vi "Procedura abilitazione potenza.vi"(9 "All Data":T3 {"MISURE ALL"."Cluster READ NI"."AI (4-20mA)"."AI 15" format="%#_6f"; "MISURE ALL"."Cluster READ NI"."AI (4-20mA)"."AI 14" format="%#_6f"; "MISURE ALL"."Cluster READ NI"."AI (4-20mA)"."AI 13" format="%#_6f"; "MISURE ALL"."Cluster READ NI"."AI (4-20mA)"."AI 11" format="%#_6f"; "MISURE ALL"."Cluster READ NI"."AI (4-20mA)"."AI 10" format="%#_6f"; "MISURE ALL"."Cluster READ NI"."AI (4-20mA)"."AI 9" format="%#_6f"; "MISURE ALL"."Cluster READ NI"."AI (4-20mA)"."AI 4" format="%#_6f"; "MISURE ALL"."Cluster READ NI"."AI (4-20mA)"."AI 12" format="%#_6f"; "MISURE ALL"."Cluster READ NI"."AI (4-20mA)"."AI 0" format="%#_6f"; "MISURE ALL"."Cluster READ NI"."AI (4-20mA)"."AI 1" format="%#_6f"; "MISURE ALL"."Cluster READ NI"."AI (4-20mA)"."AI 2" format="%#_6f"; "MISURE ALL"."Cluster READ NI"."AI (4-20mA)"."AI 3" format="%#_6f"; "MISURE ALL"."Cluster READ NI"."AI (4-20mA)"."AI 5" format="%#_6f"; "MISURE ALL"."Cluster READ NI"."AI (4-20mA)"."AI 6" format="%#_6f"; "MISURE ALL"."Cluster READ NI"."AI (4-20mA)"."AI 7" format="%#_6f"; "MISURE ALL"."Cluster READ NI"."AI (4-20mA)"."AI 8" format="%#_6f"; "MISURE ALL"."Cluster READ NI"."AI (0-10V)"."AI 31" format="%#_6f"; "MISURE ALL"."Cluster READ NI"."AI (0-10V)"."AI 30" format="%#_6f"; "MISURE ALL"."Cluster READ NI"."AI (0-10V)"."AI 29" format="%#_6f"; "MISURE ALL"."Cluster READ NI"."AI (0-10V)"."AI 28" format="%#_6f"; "MISURE ALL"."Cluster READ NI"."AI (0-10V)"."AI 27" format="%#_6f"; "MISURE ALL"."Cluster READ NI"."AI (0-10V)"."AI 26" format="%#_6f"; "MISURE ALL"."Cluster READ NI"."AI (0-10V)"."AI 25" format="%#_6f"; "MISURE ALL"."Cluster READ NI"."AI (0-10V)"."AI 24" format="%#_6f"; "MISURE ALL"."Cluster READ NI"."AI (0-10V)"."AI 23" format="%#_6f"; "MISURE ALL"."Cluster READ NI"."AI (0-10V)"."AI 22" format="%#_6f"; "MISURE ALL"."Cluster READ NI"."AI (0-10V)"."AI 21" format="%#_6f"; "MISURE ALL"."Cluster READ NI"."AI (0-10V)"."AI 20" format="%#_6f"; "MISURE ALL"."Cluster READ NI"."AI (0-10V)"."AI 19" format="%#_6f"; "MISURE ALL"."Cluster READ NI"."AI (0-10V)"."AI 18" format="%#_6f"; "MISURE ALL"."Cluster READ NI"."AI (0-10V)"."AI 17" format="%#_6f"; "MISURE ALL"."Cluster READ NI"."AI (0-10V)"."AI 16" format="%#_6f"; "MISURE ALL"."Cluster READ NI"."AI (0-10V)"."AI 15" format="%#_6f"; "MISURE ALL"."Cluster READ NI"."AI (0-10V)"."AI 14" format="%#_6f"; "MISURE ALL"."Cluster READ NI"."AI (0-10V)"."AI 13" format="%#_6f"; "MISURE ALL"."Cluster READ NI"."AI (0-10V)"."AI 11" format="%#_6f"; "MISURE ALL"."Cluster READ NI"."AI (0-10V)"."AI 10" format="%#_6f"; "MISURE ALL"."Cluster READ NI"."AI (0-10V)"."AI 9" format="%#_6f"; "MISURE ALL"."Cluster READ NI"."AI (0-10V)"."AI 4" format="%#_6f"; "MISURE ALL"."Cluster READ NI"."AI (0-10V)"."AI 12" format="%#_6f"; "MISURE ALL"."Cluster READ NI"."AI (0-10V)"."AI 0" format="%#_6f"; "MISURE ALL"."Cluster READ NI"."AI (0-10V)"."AI 1" format="%#_6f"; "MISURE ALL"."Cluster READ NI"."AI (0-10V)"."AI 2" format="%#_6f"; "MISURE ALL"."Cluster READ NI"."AI (0-10V)"."AI 3" format="%#_6f"; "MISURE ALL"."Cluster READ NI"."AI (0-10V)"."AI 5" format="%#_6f"; "MISURE ALL"."Cluster READ NI"."AI (0-10V)"."AI 6" format="%#_6f"; "MISURE ALL"."Cluster READ NI"."AI (0-10V)"."AI 7" format="%#_6f"; "MISURE ALL"."Cluster READ NI"."AI (0-10V)"."AI 8" format="%#_6f"}, 10 "Impostazioni elettriche in":T1, 11 "Stato":string) -> (0 "This VI":refnum<vi>, 2 "Fine step":bool, 3 "stato out":string)   [LabVIEW 2019]
uses:
  TypeDef/Cluster MISURE.ctl
  TypeDef/MISURE NM.ctl
  TypeDef/Cluster misure ALL.ctl
  TypeDef/Cluster NI.ctl
  cDAQ_PLC Folder/controls/StatoAO_cdaq.ctl
  cDAQ_PLC Folder/controls/statoDO_Cdaq.ctl
  TypeDef/MISURE WT.ctl
  TypeDef/ClusterRes.ctl
  TypeDef/INTERFACCIA.ctl
  TypeDef/Lista AO sistema.ctl
  TypeDef/DOinterfaccia.ctl
  cDAQ_PLC Folder/ST1200_LIST_IO/STATO PLC 1.ctl
  cDAQ_PLC Folder/ST1200_LIST_IO/Uscite PLC 1.ctl
  cDAQ_PLC Folder/controls/statoAO_plc_1.ctl
  cDAQ_PLC Folder/ST1200_LIST_IO/StatoDO_PLC_1.ctl
  SINUS PENTA SANTERNO/controls/Parametri inverter letti.ctl
  cDAQ_PLC Folder/ST1200_LIST_IO/STATO PLC 2.ctl
  cDAQ_PLC Folder/ST1200_LIST_IO/Uscite PLC 2.ctl
  cDAQ_PLC Folder/controls/statoAO_plc_2.ctl
  cDAQ_PLC Folder/ST1200_LIST_IO/StatoDO_PLC_2.ctl
  cDAQ_PLC Folder/ST1200_LIST_IO/STATO PLC 3.ctl
  cDAQ_PLC Folder/ST1200_LIST_IO/Uscite PLC 3.ctl
  cDAQ_PLC Folder/controls/statoAO_plc_3.ctl
  cDAQ_PLC Folder/ST1200_LIST_IO/StatoDO_PLC_3.ctl
  DCREG/Parametri DCREG letti.ctl
  TypeDef/Impostazioni elettriche.ctl
  TypeDef/Collegamenti_elettrici.ctl
  cDAQ_PLC Folder/cDAQ/SET ARRAY DO.ctl
  cDAQ_PLC Folder/cDAQ/SET SINGLE DO.ctl
  cDAQ_PLC Folder/cDAQ/DO List.ctl
  Stato alimentatore 1.vi
  Stato comandi freno.vi
  Global allarmi procedure.vi
panel:
  out "Stato 2":string
  out "Abilita freno":bool caption="ABILITA BANCO FRENO \\ ALIMENTATORE"
  in  "OK Button":bool
  out "String":string
  out "RESET CENTRALINA":bool caption="RESET CENTRALINA PROTEZIONI"
  out "Chiusura teleruttore":bool caption="CHIUSURA TELERUTTORE DI POTENZA"
  out "abilitazione elettroserrature":bool caption="ABILITAZIONE ELETTROSERRATURE"
  out "Verifica protezioni chiuse":bool caption="VERIFICA PROTEZIONI CHIUSE"
  # "ABILITAZIONE TELERUTTORE DI POTENZA IN CORSO. \n                               >>ATTENDI<<"
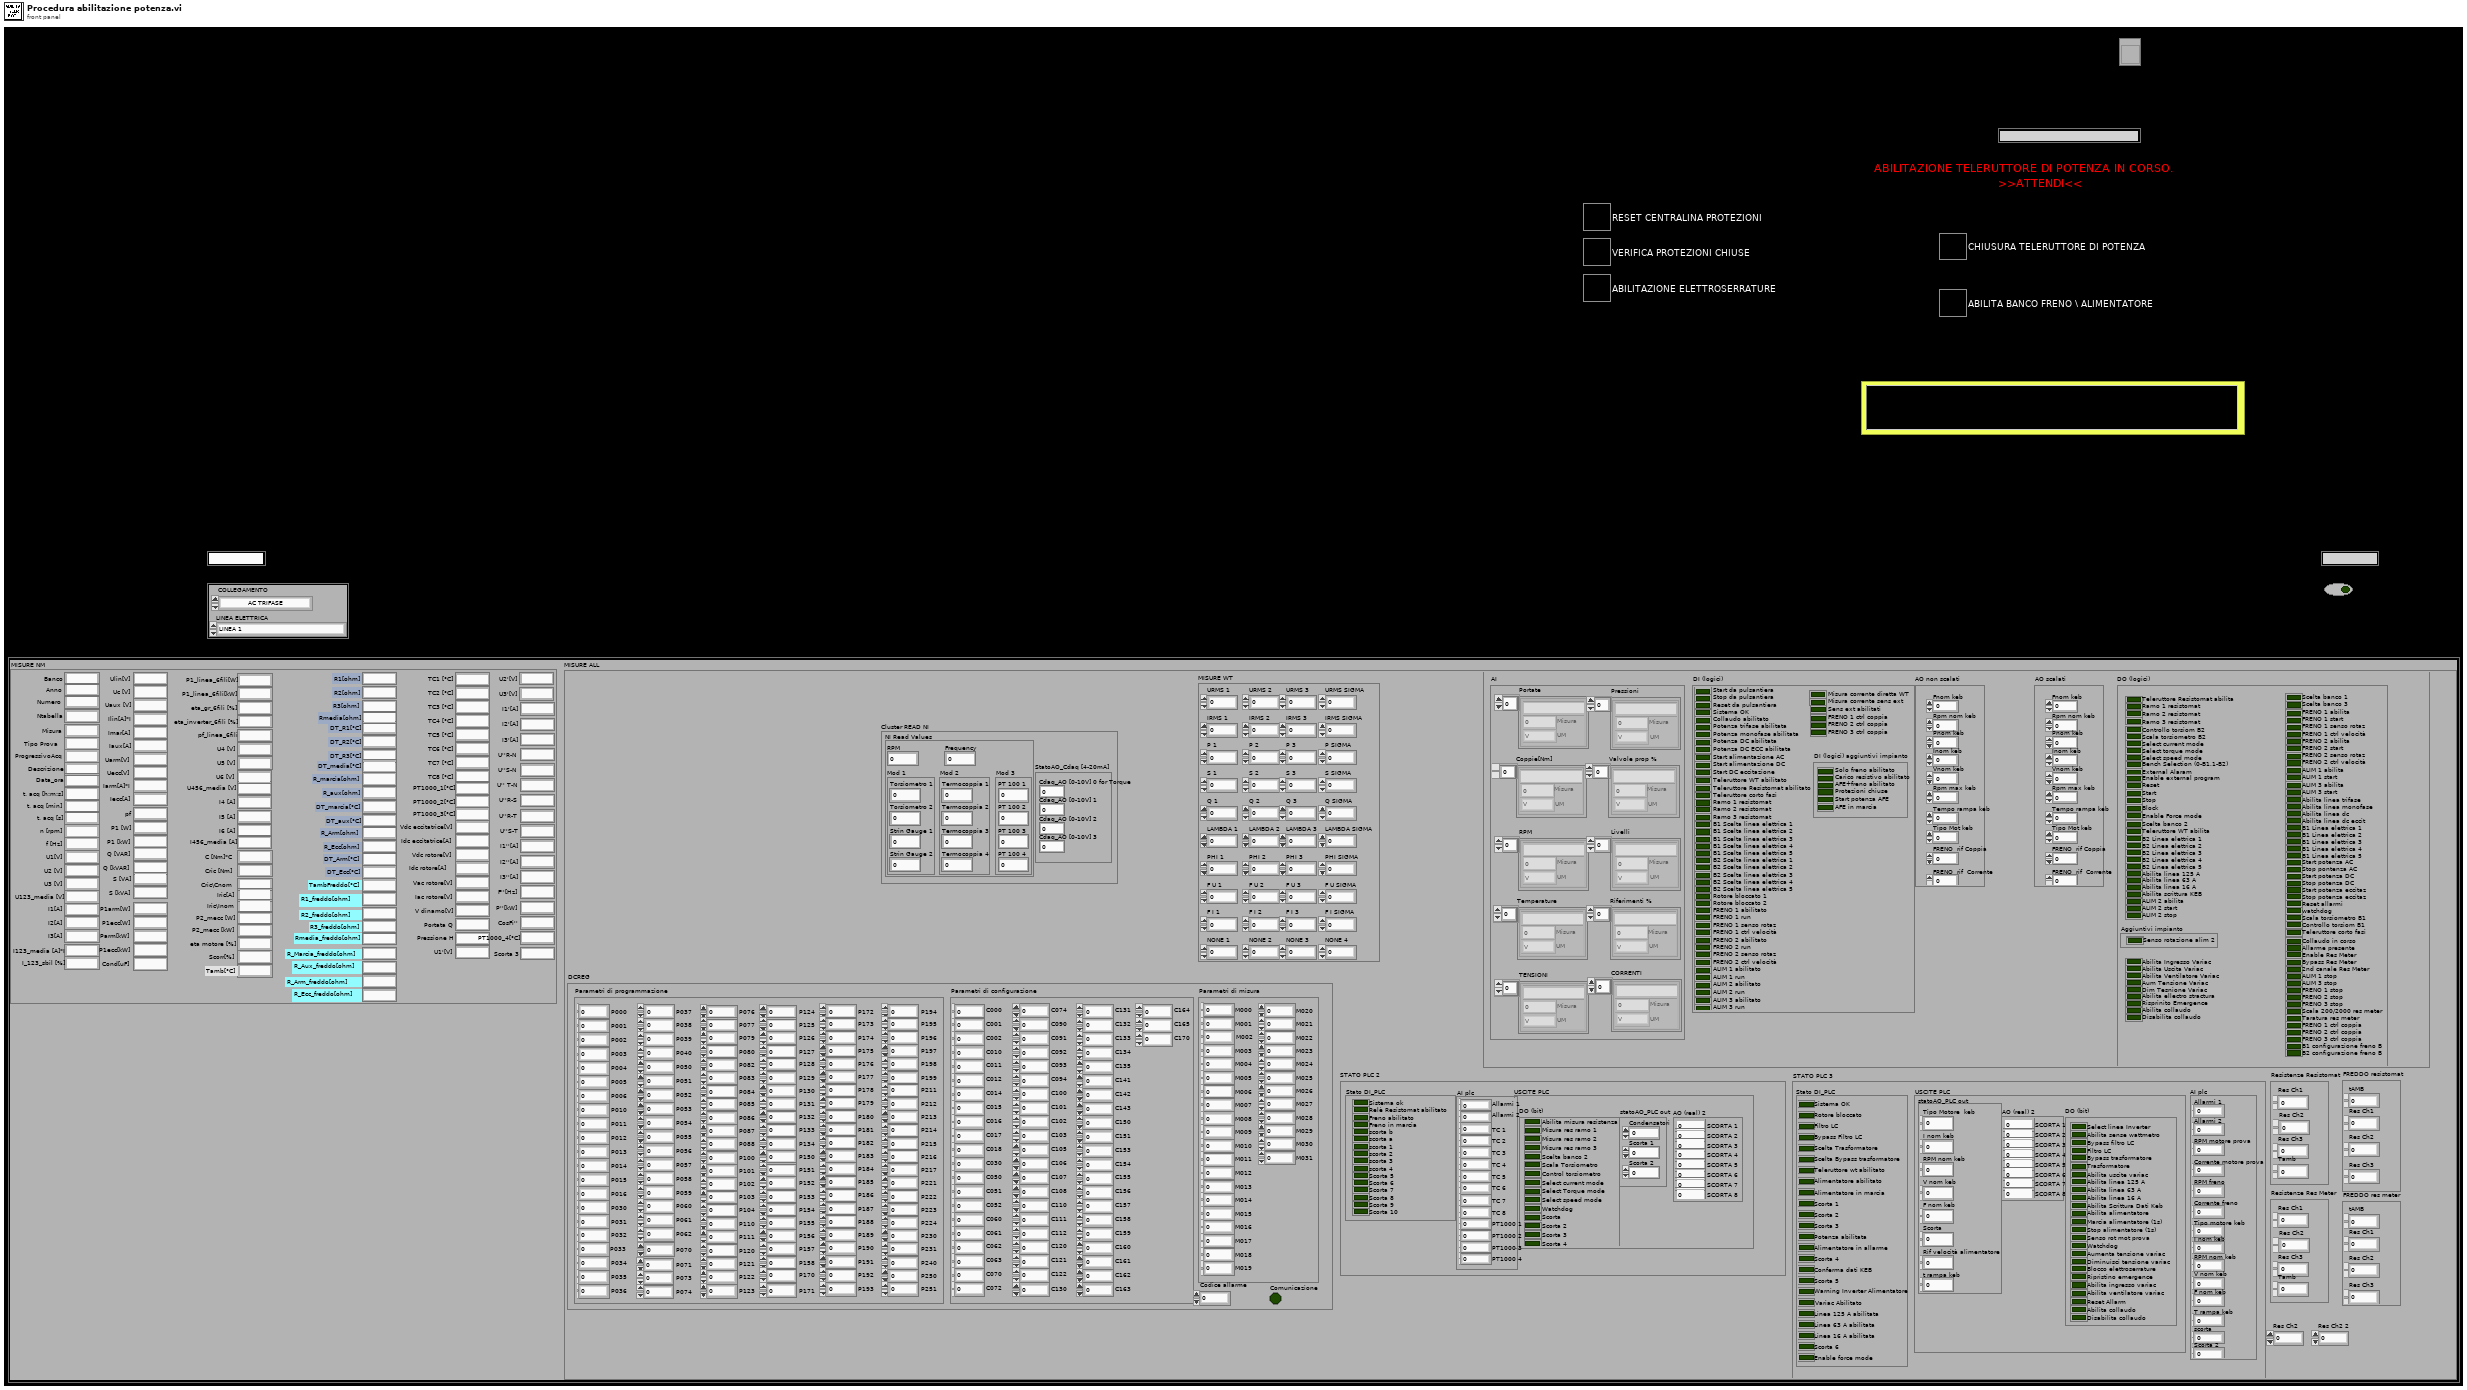
[diagram p1: front panel]
types:
  T1 = typedef "Impostazioni elettriche.ctl" = cluster{"COLLEGAMENTO":T2, "LINEA ELETTRICA":enum16{"LINEA 1", "LINEA 2", "LINEA 3", "LINEA 4", "LINEA 5"}}
  T2 = typedef "Collegamenti_elettrici.ctl" = enum16{"AC TRIFASE", "AC TRIFASE + FRENO", "AC MONOFASE", "DC CON ECCITAZIONE", "DC CON ECCITAZIONE + FRENO", "DC NO ECCITAZIONE", "DC NO ECCITAZIONE + FRENO", "FRENO TRASC + AFE", "SOLO FRENO", "CARICO RESISTIVO", "GENERICO", "SOLO ACQUISITORE", "SCORTA 4", "SCORTA 5", "SCORTA 6"}
  T3 = typedef "Cluster MISURE.ctl" = cluster{"MISURE NM":T4, "MISURE ALL":T5}
  T4 = typedef "MISURE NM.ctl" = cluster{"Banco":string, "Anno":string, "Numero":string, "Ntabella":string, "Misura":string, "Tipo Prova":string, "ProgressivoAcq":string, "Descrizione":string, "Data_ora":string, "t. acq [h:m:s]":string, "t. acq [min]":string, "t. acq [s]":string, "n [rpm]":string, "f [Hz]":string, "U1[V]":string, "U2 [V]":string, "U3 [V]":string, "U123_media [V]":string, "I1[A]":string, "I2[A]":string, "I3[A]":string, "I123_media [A]*I":string, "I_123_sbil [%]":string, "Ulin[V]":string, "Uc [V]":string, "Uaux [V]":string, "Ilin[A]*I":string, "Imar[A]":string, "Iaux[A]":string, "Uarm[V]":string, "Uecc[V]":string, "Iarm[A]*I":string, "Iecc[A]":string, "pf":string, "P1 [W]":string, "P1 [kW]":string, "Q [VAR]":string, "Q [kVAR]":string, "S [VA]":string, "S [kVA]":string, "P1arm[W]":string, "P1ecc[W]":string, "Parm[kW]":string, "P1ecc[kW]":string, "Cond[uF]":string, "P1_linea_6fili[W]":string, "P1_linea_6fili[kW]":string, "eta_gr_6fili [%]":string, "eta_inverter_6fili [%]":string, "pf_linea_6fili":string, "U4 [V]":string, "U5 [V]":string, "U6 [V]":string, "U456_media [V]":string, "I4 [A]":string, "I5 [A]":string, "I6 [A]":string, "I456_media [A]":string, "C [Nm]*C":string, "Cric [Nm]":string, "Cric\\Cnom":string, "Iric[A]":string, "Iric\\Inom":string, "P2_mecc [W]":string, "P2_mecc [kW]":string, "eta motore [%]":string, "Scorr[%]":string, "Tamb[°C]":string, "R1[ohm]":string, "R2[ohm]":string, "R3[ohm]":string, "Rmedia[ohm]":string, "DT_R1[°C]":string, "DT_R2[°C]":string, "DT_R3[°C]":string, "DT_media[°C]":string, "R_marcia[ohm]":string, "R_aux[ohm]":string, "DT_marcia[°C]":string, "DT_aux[°C]":string, "R_Arm[ohm]":string, "R_Ecc[ohm]":string, "DT_Arm[°C]":string, "DT_Ecc[°C]":string, "TambFreddo[°C]":string, "R1_freddo[ohm]":string, "R2_freddo[ohm]":string, "R3_freddo[ohm]":string, "Rmedia_freddo[ohm]":string, "R_Marcia_freddo[ohm]":string, "R_Aux_freddo[ohm]":string, "R_Arm_freddo[ohm]":string, "R_Ecc_freddo[ohm]":string, "TC1 [°C]":string, "TC2 [°C]":string, "TC3 [°C]":string, "TC4 [°C]":string, "TC5 [°C]":string, "TC6 [°C]":string, "TC7 [°C]":string, "TC8 [°C]":string, "PT1000_1[°C]":string, "PT1000_2[°C]":string, "PT1000_3[°C]":string, "Vdc eccitatrice[V]":string, "Idc eccitatrice[A]":string, "Vdc rotore[V]":string, "Idc rotore[A]":string, "Vac rotore[V]":string, "Iac rotore[V]":string, "V dinamo[V]":string, "Portata Q":string, "Pressione H":string, "U1'[V]":string, "U2'[V]":string, "U3'[V]":string, "I1'[A]":string, "I2'[A]":string, "I3'[A]":string, "U''R-N":string, "U''S-N":string, "U'' T-N":string, "U''R-S":string, "U''R-T":string, "U''S-T":string, "I1''[A]":string, "I2''[A]":string, "I3''[A]":string, "F''[Hz]":string, "P''[kW]":string, "CosFi''":string, "PT1000_4[°C]":string, "Scorta 3":string}
  T5 = typedef "Cluster misure ALL.ctl" = cluster{"Cluster READ NI":T6, "MISURE WT":T9, "Resistenze Resistomat":T10, "INTERFACCIA":T11, "FREDDO resistomat":cluster{"Res Ch1":dbl, "Res Ch2":dbl, "tAMB":dbl, "Res Ch3":dbl}, "STATO PLC 1":T16, "Res Ch2":dbl, "Res Ch2 2":dbl, "FREDDO res meter":cluster{"Res Ch1":dbl, "Res Ch2":dbl, "tAMB":dbl, "Res Ch3":dbl}, "Resistenze Res Meter":T10, "READ SINUS PENTA":T20, "STATO PLC 2":T21, "STATO PLC 3":T25, "DCREG":T29}
  T6 = typedef "Cluster NI.ctl" = cluster{"AI (0-10V)":cluster{"AI 0":dbl, "AI 1":dbl, "AI 2":dbl, "AI 3":dbl, "AI 4":dbl, "AI 5":dbl, "AI 6":dbl, "AI 7":dbl, "AI 8":dbl, "AI 9":dbl, "AI 10":dbl, "AI 11":dbl, "AI 12":dbl, "AI 13":dbl, "AI 14":dbl, "AI 15":dbl, "AI 16":dbl, "AI 17":dbl, "AI 18":dbl, "AI 19":dbl, "AI 20":dbl, "AI 21":dbl, "AI 22":dbl, "AI 23":dbl, "AI 24":dbl, "AI 25":dbl, "AI 26":dbl, "AI 27":dbl, "AI 28":dbl, "AI 29":dbl, "AI 30":dbl, "AI 31":dbl}, "StatoAO_Cdaq[0-10V]":cluster{"AO 1":dbl, "AO 2":dbl, "AO 3":dbl, "AO 4":dbl}, "Contatori [rpm]":cluster{"RPM 1":dbl, "RPM 2":dbl}, "StatoAO_Cdaq [4-20mA]":T7, "StatoDO_Cdaq":T8, "DI":cluster{"Scorta 0":bool, "Scorta 1":bool, "Scorta 2":bool, "Scorta 3":bool, "Scorta 4":bool, "Scorta 5":bool, "Scorta 6":bool, "Scorta 7":bool, "Scorta 8":bool, "Scorta 9":bool, "Scorta 10":bool, "Scorta 11":bool, "Scorta 12":bool, "Scorta 13":bool, "Scorta 14":bool, "Scorta 15":bool, "Scorta 16":bool, "Scorta 17":bool, "Scorta 18":bool, "Scorta 19":bool, "Scorta 20":bool, "Scorta 21":bool, "Scorta 22":bool, "Scorta 23":bool, "Scorta 24":bool, "Scorta 25":bool, "Scorta 26":bool, "Scorta 27":bool, "Scorta 28":bool, "Scorta 29":bool, "Scorta 30":bool, "Scorta 31":bool}, "AI (4-20mA)":cluster{"AI 0":dbl, "AI 1":dbl, "AI 2":dbl, "AI 3":dbl, "AI 4":dbl, "AI 5":dbl, "AI 6":dbl, "AI 7":dbl, "AI 8":dbl, "AI 9":dbl, "AI 10":dbl, "AI 11":dbl, "AI 12":dbl, "AI 13":dbl, "AI 14":dbl, "AI 15":dbl}, "TC [°C]":cluster{"tc 1":dbl, "tc 2":dbl, "tc 3":dbl, "tc 4":dbl}, "NI Read Values":cluster{"RPM":dbl, "Frequency":dbl, "Mod 1":cluster{"Torsiometro 1":dbl, "Torsiometro 2":dbl, "Strin Gauge 1":dbl, "Strin Gauge 2":dbl}, "Mod 2":cluster{"Termocoppia 1":dbl, "Termocoppia 2":dbl, "Termocoppia 3":dbl, "Termocoppia 4":dbl}, "Mod 3":cluster{"PT 100 1":dbl, "PT 100 2":dbl, "PT 100 3":dbl, "PT 100 4":dbl}}}
  T7 = typedef "StatoAO_cdaq.ctl" = cluster{"Cdaq_AO [0-10V] 0 for Torque":dbl, "Cdaq_AO [0-10V] 1":dbl, "Cdaq_AO [0-10V] 2":dbl, "Cdaq_AO [0-10V] 3":dbl}
  T8 = typedef "statoDO_Cdaq.ctl" = cluster{"Scorta 0":bool, "Scorta 1":bool, "Scorta 2":bool, "Scorta 3":bool, "Scorta 4":bool, "Scorta 5":bool, "Scorta 6":bool, "Scorta 7":bool, "Scorta 8":bool, "Scorta 9":bool, "Scorta 10":bool, "Scorta 11":bool, "Scorta 12":bool, "Scorta 13":bool, "Scorta 14":bool, "Scorta 15":bool, "Scorta 16":bool, "Scorta 17":bool, "Scorta 18":bool, "Scorta 19":bool, "Scorta 20":bool, "Scorta 21":bool, "Scorta 22":bool, "Scorta 23":bool, "Scorta 24":bool, "Scorta 25":bool, "Scorta 26":bool, "Scorta 27":bool, "Scorta 28":bool, "Scorta 29":bool, "Scorta 30":bool, "Scorta 31":bool}
  T9 = typedef "MISURE WT.ctl" = cluster{"URMS 1":dbl, "IRMS 1":dbl, "P 1":dbl, "S 1":dbl, "Q 1":dbl, "LAMBDA 1":dbl, "PHI 1":dbl, "F U 1":dbl, "F I 1":dbl, "NONE 1":dbl, "URMS 2":dbl, "IRMS 2":dbl, "P 2":dbl, "S 2":dbl, "Q 2":dbl, "LAMBDA 2":dbl, "PHI 2":dbl, "F U 2":dbl, "F I 2":dbl, "NONE 2":dbl, "URMS 3":dbl, "IRMS 3":dbl, "P 3":dbl, "S 3":dbl, "Q 3":dbl, "LAMBDA 3":dbl, "PHI 3":dbl, "F U 3":dbl, "F I 3":dbl, "NONE 3":dbl, "URMS SIGMA":dbl, "IRMS SIGMA":dbl, "P SIGMA":dbl, "S SIGMA":dbl, "Q SIGMA":dbl, "LAMBDA SIGMA":dbl, "PHI SIGMA":dbl, "F U SIGMA":dbl, "F I SIGMA":dbl, "NONE 4":dbl}
  T10 = typedef "ClusterRes.ctl" = cluster{"Res Ch1":dbl, "Res Ch2":dbl, "Res Ch3":dbl, "Tamb":dbl}
  T11 = typedef "INTERFACCIA.ctl" = cluster{"AI":cluster{"Portate":T12[], "Pressioni":T12[], "Coppie[Nm]":T12[], "Valvole prop %":T12[], "RPM":T12[], "Livelli":T12[], "Temperature":T12[], "Riferimenti %":T12[], "TENSIONI":T12[], "CORRENTI":T12[]}, "DI (logici)":cluster{"Start da pulsantiera":bool, "Stop da pulsantiera":bool, "Reset da pulsantiera":bool, "Sistema OK":bool, "Collaudo abilitato":bool, "Potenza trifase abilitata":bool, "Potenza monofase abilitata":bool, "Potenza DC abilitata":bool, "Potenza DC ECC abilitata":bool, "Start alimentazione AC":bool, "Start alimentazione DC":bool, "Start DC eccitazione":bool, "Teleruttore WT abilitato":bool, "Teleruttore Resistomat abilitato":bool, "Teleruttore corto fasi":bool, "Ramo 1 resistomat":bool, "Ramo 2 resistomat":bool, "Ramo 3 resistomat":bool, "B1 Scelta linea elettrica 1":bool, "B1 Scelta linea elettrica 2":bool, "B1 Scelta linea elettrica 3":bool, "B1 Scelta linea elettrica 4":bool, "B1 Scelta linea elettrica 5":bool, "B2 Scelta linea elettrica 1":bool, "B2 Scelta linea elettrica 2":bool, "B2 Scelta linea elettrica 3":bool, "B2 Scelta linea elettrica 4":bool, "B2 Scelta linea elettrica 5":bool, "Rotore bloccato 1":bool, "Rotore bloccato 2":bool, "FRENO 1 abilitato":bool, "FRENO 1 run":bool, "FRENO 1 senso rotaz":bool, "FRENO 1 ctrl velocità":bool, "FRENO 2 abilitato":bool, "FRENO 2 run":bool, "FRENO 2 senso rotaz":bool, "FRENO 2 ctrl velocità":bool, "ALIM 1 abilitato":bool, "ALIM 1 run":bool, "ALIM 2 abilitato":bool, "ALIM 2 run":bool, "ALIM 3 abilitato":bool, "ALIM 3 run":bool, "FRENO 1 ctrl coppia":bool, "FRENO 2 ctrl coppia":bool, "FRENO 3 ctrl coppia":bool, "DI (logici) aggiuntivi impianto":cluster{"Solo freno abilitato":bool, "Carico resistivo abilitato":bool, "AFE+freno abilitato":bool, "Protezioni chiuse":bool, "Start potenza AFE":bool, "AFE in marcia":bool}, "Misura corrente diretta WT":bool, "Misura corrente sens ext":bool, "Sens ext abilitati":bool}, "AO non scalati":T14, "AO scalati":T14, "DO (logici)":T15}
  T12 = typedef "ClusterMisura_e_Unità_INPUT.ctl" = cluster{"Misura":dbl, "UM":T13, "Descrizione":string}
  T13 = typedef "UnitàMisura.ctl" = enum16{"V", "mA", "Bar", "RPM", "m3/s", "m3/min", "m3/h", "l/s", "l/min", "in3/min", "ft3/min", "gpm", "igpm", "igph", "%", "°C", "m", "Nm", "A"}
  T14 = typedef "Lista AO sistema.ctl" = cluster{"FRENO1 rif vel":dbl, "FRENO1 rif Coppia":dbl, "FRENO2 rif vel":dbl, "FRENO2 rif Coppia":dbl, "ALIM1 rif V":dbl, "ALIM1 rif F":dbl, "ALIM2 rif V":dbl, "ALIM2 rif F":dbl, "ALIM3 rif V":dbl, "ALIM3 rif F":dbl, "Fnom keb":dbl, "Rpm nom keb":dbl, "Pnom keb":dbl, "Inom keb":dbl, "Vnom keb":dbl, "Rpm max keb":dbl, "Tempo rampa keb":dbl, "Tipo Mot keb":dbl, "FRENO  rif Coppia ":dbl, "FRENO  rif  Corrente":dbl}
  T15 = typedef "DOinterfaccia.ctl" = cluster{"Scelta banco 1":bool, "Scelta banco 2":bool, "Scelta banco 3":bool, "FRENO 1 abilita":bool, "FRENO 1 start":bool, "FRENO 1 senso rotaz":bool, "FRENO 1 ctrl velocità":bool, "FRENO 2 abilita":bool, "FRENO 2 start":bool, "FRENO 2 senso rotaz":bool, "FRENO 2 ctrl velocità":bool, "ALIM 1 abilita":bool, "ALIM 1 start":bool, "ALIM 2 abilita":bool, "ALIM 2 start":bool, "ALIM 3 abilita":bool, "ALIM 3 start":bool, "Abilita linea trifase":bool, "Abilita linea monofase":bool, "Abilita linea dc":bool, "Abilita linea dc eccit":bool, "B1 Linea elettrica 1":bool, "B1 Linea elettrica 2":bool, "B1 Linea elettrica 3":bool, "B1 Linea elettrica 4":bool, "B1 Linea elettrica 5":bool, "B2 Linea elettrica 1":bool, "B2 Linea elettrica 2":bool, "B2 Linea elettrica 3":bool, "B2 Linea elettrica 4":bool, "B2 Linea elettrica 5":bool, "Start potenza AC":bool, "Stop pontenza AC":bool, "Start potenza DC":bool, "Stop potenza DC":bool, "Start potenza eccitaz":bool, "Stop potenza eccitaz":bool, "Reset allarmi":bool, "watchdog":bool, "Scala torsiometro B1":bool, "Controllo torsiom B1":bool, "Scala torsiometro B2":bool, "Controllo torsiom B2":bool, "Teleruttore WT abilita":bool, "Teleruttore Resistomat abilita":bool, "Teleruttore corto fasi":bool, "Ramo 1 resistomat":bool, "Ramo 2 resistomat":bool, "Ramo 3 resistomat":bool, "Collaudo in corso":bool, "Allarme presente":bool, "Enable Res Meter":bool, "Bypass Res Meter":bool, "2nd canale Res Meter":bool, "Scala 200/2000 res meter":bool, "Taratura res meter":bool, "FRENO 1 ctrl coppia":bool, "FRENO 2 ctrl coppia":bool, "FRENO 3 ctrl coppia":bool, "Aggiuntivi impianto":cluster{"Senso rotazione alim 1":bool, "Senso rotazione alim 2":bool}, "ALIM 1 stop":bool, "ALIM 2 stop":bool, "ALIM 3 stop":bool, "FRENO 1 stop":bool, "FRENO 2 stop":bool, "FRENO 3 stop":bool, "B1 configurazione freno B":bool, "B2 configurazione freno B":bool, "Abilita scrittura KEB":bool, "Bench Selection (0-B1,1-B2)":bool, "Select current mode":bool, "Select torque mode":bool, "Select speed mode":bool, "Start":bool, "Stop":bool, "Block":bool, "Enable Force mode":bool, "Abilita linea 125 A":bool, "Abilita linea 63 A":bool, "Abilita linea 16 A":bool, "Aum Tensione Variac":bool, "Dim Tesnione Variac":bool, "Abilita ellectro stractura":bool, "Risprinito Emergence":bool, "Abilita collaudo":bool, "Disabilita collaudo":bool, "External Alaram":bool, "Enable external program":bool, "Reset":bool, "Abilita Ingresso Variac":bool, "Abilita Ventilatore Variac":bool, "Abilita Uscita Variac ":bool}
  T16 = typedef "STATO PLC 1.ctl" = cluster{"USCITE PLC":T17, "Stato DI_PLC":cluster{"Sistema OK":bool, "Rotore bloccato":bool, "Scorta 1":bool, "Prova diretto inverter":bool, "Prova con filtro LC":bool, "Teleruttore WT abilitato":bool, "Alim sinus penta abilitato":bool, "Alim sinus penta in marcia":bool, "Freno abilitato":bool, "Freno in marcia":bool, "Senso rotazione freno":bool, "Potenza abilitata":bool, "Scorta 3":bool, "Scorta 4":bool, "scorta 5":bool, "scorta 6":bool}, "AI plc":cluster{"Allarmi 1":dbl, "Allarmi 2":dbl, "Scorta 1":dbl, "Scorta 2":dbl, "RPM mot prova":dbl, "I mot prova":dbl, "RPM freno":dbl, "I freno":dbl, "Scorta 3":dbl, "Scorta 4":dbl}}
  T17 = typedef "Uscite PLC 1.ctl" = cluster{"AO (real) 2":cluster{"SCORTA 1":dbl, "SCORTA 2":dbl, "SCORTA 3":dbl, "SCORTA 4":dbl, "SCORTA 5":dbl, "SCORTA 6":dbl, "SCORTA 7":dbl, "SCORTA 8":dbl}, "statoAO_PLC out":T18, "DO (bit)":T19}
  T18 = typedef "statoAO_plc_1.ctl" = cluster{"Rif Lim coppia freno [%]":dbl, "Rif rpm freno [%]":dbl, "Rif coppia freno [%]":dbl, "Rif V alimentatore [%]":dbl, "Rif F alimentatore [%]":dbl}
  T19 = typedef "StatoDO_PLC_1.ctl" = cluster{"Scelta banco 1":bool, "Set dati motore freno 2":bool, "Diretto inverter":bool, "Filtro LC":bool, "Marcia ALIM (1s)":bool, "Marcia FRENO (1s)":bool, "Stop AFE (1s)":bool, "Stop freno (1s)":bool, "Reset allarmi":bool, "Watchdog":bool, "Senso rotazione":bool, "Abilita collaudo (1s)":bool, "Disabilita collaudo (1s)":bool, "Abilitazione ALIM":bool, "Abilitazione FRENO":bool, "Teleruttore WT":bool, "Senso rot motore prova":bool, "Scorta 7":bool, "Scorta 8":bool, "Scorta 9":bool, "Scorta 10":bool, "Scorta 11":bool, "Scorta 12":bool, "Scorta 13":bool}
  T20 = typedef "Parametri inverter letti.ctl" = cluster{"Menù Misure motore (M000-M030)":cluster{"Rif vel a regime (int)":u16, "Rif vel a regime (dec)":u16, "Rif vel dopo rampe (int)":u16, "Rif vel dopo rampe (dec)":u16, "RPM motore (int)":u16, "RPM motore (dec)":u16, "FREQout inverter":u16, "Rif coppia a regime(Nm)":u16, "Richiesta di coppia (Nm)":u16, "Coppia generata dal motore(Nm)":u16, "Rif coppia a regime(%)":u16, "Richiesta di coppia (%)":u16, "Coppia generata dal motore(%)":u16, "Coppia max richiesta prima delle rampe(Nm)":u16, "Coppia max richiesta dopo le rampe(Nm)":u16, "Limite di velocità prima delle rampe":u16, "Limite di velocità dopo le rampe":u16, "Coppia max richiesta prima delle rampe(%)":u16, "Coppia max richiesta dopo le rampe(%)":u16, "Rif di flusso":u16, "Corrente di uscita":u16, "Capacità termica del motore":u16, "Tensione di uscita":u16, "Potenza di uscita":u16, "Energia consumata (LSword)":u16, "Energia consumata (MSword)":u16, "Tensione bus DC":u16, "Tensione di rete":u16}, "Menù regolatore PID (M018-M024)":cluster{"Rif PID a regime(%)":u16, "Rif pid dopo rampe(%)":u16, "Retroazione del pid(%)":u16, "Errore del pid(%)":u16, "uscita del pid(%)":u16, "Rif del pid dopo le rampe":u16, "Retroazione del pid":u16}, "Menù ingressi digitali (M031-M036)":cluster{"Ingressi digitali ritardati":u16, "Ingressi digitali istantanei":u16, "Moresettiera comando loc":u16, "Morsett comando da seriale":u16, "Morsett comando bus di campo":u16, "Ing dig ausiliari da morsettiera":u16, "Ing dig ausiliari da seriale":u16}, "Menù riferimenti (M037-M051)":cluster{"Rif analog est REF":u16, "Rif analog est AIN1":u16, "Rif analog est AIN2":u16, "Rif analog est XAIN4":u16, "Rif analog est XAIN5":u16, "Rif velocità da seriale(int)":u16, "Rif velocità bus di campo(int)":u16, "Rif coppia da seriale":u16, "Rif coppia bus di campo":u16, "Rif del PID da seriale":u16, "Rif del PID da bus di campo":u16, "Retroazione del PID da seriale":u16, "Retroazione del PIDda bus di campo":u16, "Rif da encoder":u16, "Rif in frequenza":u16, "Rif velocità da seriale(dec)":u16, "Rif velocità bus di campo(dec)":u16}, "Menù rampe (P009-P033)":cluster{"Tempo di dec rampa di vel 1":u16, "Tempo di acc rampa di vel 2":u16, "Tempo di dec rampa di vel 2":u16, "Tempo di acc rampa di vel 1":u16, "Unità di mis tempi rampe vel 1/2":u16, "Tempo di acc rampa di vel 3":u16, "Tempo di dec rampa di vel 3":u16, "Tempo di acc rampa di vel 4":u16, "Tempo di dec rampa di vel 4":u16, "Unità di mis tempi rampe vel 3/4":u16, "Selettore arrottondam rampe":u16, "Tempo di arrotond iniz rampa acc":u16, "Tempo di arrotond finale rampa acc":u16, "Tempo di arrotond iniz rampa dec":u16, "Tempo di rampa di salita rif coppia":u16, "Tempo di rampa di discesa rif coppia":u16, "Unità di misura rampa coppia":u16, "Tempo rampa acc marcia jog":u16, "Tempo rampa dec marcia jog":u16, "Reset acc ai cambi pendenza":u16, "rampa di acc in fire mode":u16, "rampa di dec in fire mode":u16, "Tempo di arrotond finale rampa dec":u16}, "Menù controllo motore(C008-C128)":cluster{"Numero motori configurati":u16, "Tipo algoritmo di controllo Mot1":u16, "Tipo rif Mot1":u16, "Tensione nominale rete":u16, "Retroaz di vel da encoder Mot1":u16, "Tipo curva V/f Mot1":u16, "Rotazione delle fasi Mot1":u16, "Freq nominale del motore Mot1":u16, "RPM nominali del motore Mot1":u16, "Potenza nominale del motore Mot1":u16, "Corrente nominale del motore Mot1":u16, "Tensione nominale del motore mot1":u16, "Potenza a vuoto del motore Mot1":u16, "Corrente a vuoto del motore Mot1":u16, "Resistenza statorica del motore Mot1":u16, "Induttanza di dispersione Mot1":u16, "Induttanza mutua motore":u16, "Costante di tempo rotorica":u16, "Costante di tempo filtro pb":u16, "Velocità minima motore":u16, "Velocità massima motore":u16}, "Menù configurazione PID":cluster{"Selezione riferimento n.1":u16, "Selezione retroazione n.1":u16, "Modalità di fuzionamento PID":u16, "Termine derivativo calcolato su err o mis":u16, "Proporz moltiplica deriv e integrale":u16, "Azione del PID":u16}, "ID":dbl, "Menù uscite digitali":cluster{"MDO4 Inverter pronto":u16}, "Fcarrier":cluster{"Fcarrier Min (Hz)":u16, "Fcarrier Max (Hz)":u16}, "stato inverter M089":dbl, "Riferimenti":cluster{"Rif tensione":u16, "Rif velocità":u16}, "Comunicazione":bool, "Modalità stop":dbl}
  T21 = typedef "STATO PLC 2.ctl" = cluster{"USCITE PLC":T22, "Stato DI_PLC":cluster{"Sistema ok":bool, "Relè Resistomat abilitato":bool, "Freno abilitato":bool, "Freno in marcia":bool, "scorta b":bool, "scorta a":bool, "scorta 1":bool, "scorta 2":bool, "scorta 3":bool, "scorta 4":bool, "Scorta 5":bool, "Scorta 6":bool, "Scorta 7":bool, "Scorta 8":bool, "Scorta 9":bool, "Scorta 10":bool}, "AI plc":cluster{"Allarmi 1":dbl, "Allarmi 2":dbl, "TC 1":dbl, "TC 2":dbl, "TC 3":dbl, "TC 4":dbl, "TC 5":dbl, "TC 6":dbl, "TC 7":dbl, "TC 8":dbl, "PT1000 1":dbl, "PT1000 2":dbl, "PT1000 3":dbl, "PT1000 4":dbl}}
  T22 = typedef "Uscite PLC 2.ctl" = cluster{"AO (real) 2":cluster{"SCORTA 1":dbl, "SCORTA 2":dbl, "SCORTA 3":dbl, "SCORTA 4":dbl, "SCORTA 5":dbl, "SCORTA 6":dbl, "SCORTA 7":dbl, "SCORTA 8":dbl}, "statoAO_PLC out":T23, "DO (bit)":T24}
  T23 = typedef "statoAO_plc_2.ctl" = cluster{"Condensatori":dbl, "Scorta 1":dbl, "Scorta 2":dbl}
  T24 = typedef "StatoDO_PLC_2.ctl" = cluster{"Relè misura resistomat":bool, "Misura res ramo 1":bool, "Misura res ramo 2":bool, "Misura res ramo 3":bool, "Scelta banco 2":bool, "Scala Torsiometro":bool, "Ctrl torsiometro":bool, "Select current mode":bool, "Select Torque mode":bool, "Select speed mode":bool, "Watchdog":bool, "Scorta":bool, "Scorta 2":bool, "Scorta 3":bool, "Scorta 4":bool, "Scorta 5":bool, "Bench selection":bool, "External alarm":bool, "Enable external program":bool, "Reset allarmi":bool, "Start":bool, "Stop":bool, "Block":bool, "Scorta 6":bool}
  T25 = typedef "STATO PLC 3.ctl" = cluster{"USCITE PLC":T26, "Stato DI_PLC":cluster{"Sistema OK":bool, "Rotore bloccato":bool, "Filtro LC":bool, "Bypass Filtro LC":bool, "Scelta Trasformatore":bool, "Scelta Bypass trasformatore":bool, "Teleruttore wt abilitato":bool, "Alimentatore abilitato":bool, "Alimentatore in marcia":bool, "Scorta 1":bool, "Scorta 2":bool, "Scorta 3":bool, "Potenza abilitata":bool, "Alimentatore in allarme":bool, "Scorta 4":bool, "Conferma dati KEB":bool, "Scorta 5":bool, "Warning Inverter Alimentatore":bool, "Variac Abilitato":bool, "Linea 125 A abilitata":bool, "Linea 63 A abilitata":bool, "Linea 16 A abilitata":bool, "Scorta 6":bool, "Enable force mode":bool}, "AI plc":cluster{"Allarmi 1":dbl, "Allarmi 2":dbl, "RPM motore prova":dbl, "Corrente motore prova":dbl, "RPM freno":dbl, "Corrente freno":dbl, "Tipo motore keb":dbl, "I nom keb":dbl, "RPM nom keb":dbl, "V nom keb":dbl, "F nom keb":dbl, "T rampa keb":dbl, "scorta":dbl, "Scorta 2":dbl}}
  T26 = typedef "Uscite PLC 3.ctl" = cluster{"AO (real) 2":cluster{"SCORTA 1":dbl, "SCORTA 2":dbl, "SCORTA 3":dbl, "SCORTA 4":dbl, "SCORTA 5":dbl, "SCORTA 6":dbl, "SCORTA 7":dbl, "SCORTA 8":dbl}, "statoAO_PLC out":T27, "DO (bit)":T28}
  T27 = typedef "statoAO_plc_3.ctl" = cluster{"Rif velocità alimentatore":dbl, "Scorta":dbl, "Tipo Motore  keb":dbl, "I nom keb":dbl, "RPM nom keb":dbl, "V nom keb":dbl, "F nom keb":dbl, "t rampa keb":dbl}
  T28 = typedef "StatoDO_PLC_3.ctl" = cluster{"Select linea Inverter":bool, "Abilita sense wattmetro":bool, "Bypass filtro LC":bool, "Filtro LC":bool, "Bypass trasformatore":bool, "Trasformatore":bool, "Abilita uscite variac":bool, "Abilita linea 125 A":bool, "Abilita linea 63 A":bool, "Abilita linea 16 A":bool, "Abilita Scrittura Dati Keb":bool, "Abilita alimentatore":bool, "Marcia alimentatore (1s)":bool, "Stop alimentatore (1s)":bool, "Senso rot mot prova":bool, "Watchdog":bool, "Aumenta tensione variac":bool, "Diminuisci tensione variac ":bool, "Blocco elettroserrature":bool, "Ripristino emergence":bool, "Abilita ingresso variac":bool, "Abilita ventilatore variac":bool, "Reset Allarm":bool, "Scorta 1":bool, "Scorta 2":bool, "Scorta 3":bool, "Scorta 4":bool, "Scorta 5":bool, "Scorta 6":bool, "Scorta 7":bool, "Scorta 8":bool, "Scorta 9":bool, "Abilita collaudo":bool, "Disabilita collaudo ":bool, "Scorta 10":bool, "Scorta 11":bool, "Scorta 12":bool, "Scorta 13":bool, "Scorta 14":bool, "Scorta 15":bool}
  T29 = typedef "Parametri DCREG letti.ctl" = cluster{"Parametri di misura":cluster{"M000":dbl, "M001":dbl, "M002":dbl, "M003":dbl, "M004":dbl, "M005":dbl, "M006":dbl, "M007":dbl, "M008":dbl, "M009":dbl, "M010":dbl, "M011":dbl, "M012":dbl, "M013":dbl, "M014":dbl, "M015":dbl, "M016":dbl, "M017":dbl, "M018":dbl, "M019":dbl, "M020":dbl, "M021":dbl, "M022":dbl, "M023":dbl, "M024":dbl, "M025":dbl, "M026":dbl, "M027":dbl, "M028":dbl, "M029":dbl, "M030":dbl, "M031":dbl}, "Parametri di programmazione":cluster{"P000":dbl, "P001":dbl, "P002":dbl, "P003":dbl, "P004":dbl, "P005":dbl, "P006":dbl, "P010":dbl, "P011":dbl, "P012":dbl, "P013":dbl, "P014":dbl, "P015":dbl, "P016":dbl, "P030":dbl, "P031":dbl, "P032":dbl, "P033":dbl, "P034":dbl, "P035":dbl, "P036":dbl, "P037":dbl, "P038":dbl, "P039":dbl, "P040":dbl, "P050":dbl, "P051":dbl, "P052":dbl, "P053":dbl, "P054":dbl, "P055":dbl, "P056":dbl, "P057":dbl, "P058":dbl, "P059":dbl, "P060":dbl, "P061":dbl, "P062":dbl, "P070":dbl, "P071":dbl, "P073":dbl, "P074":dbl, "P076":dbl, "P077":dbl, "P079":dbl, "P080":dbl, "P082":dbl, "P083":dbl, "P084":dbl, "P085":dbl, "P086":dbl, "P087":dbl, "P088":dbl, "P100":dbl, "P101":dbl, "P102":dbl, "P103":dbl, "P104":dbl, "P110":dbl, "P111":dbl, "P120":dbl, "P121":dbl, "P122":dbl, "P123":dbl, "P124":dbl, "P125":dbl, "P126":dbl, "P127":dbl, "P128":dbl, "P129":dbl, "P130":dbl, "P131":dbl, "P132":dbl, "P133":dbl, "P134":dbl, "P150":dbl, "P151":dbl, "P152":dbl, "P153":dbl, "P154":dbl, "P155":dbl, "P156":dbl, "P157":dbl, "P158":dbl, "P170":dbl, "P171":dbl, "P172":dbl, "P173":dbl, "P174":dbl, "P175":dbl, "P176":dbl, "P177":dbl, "P178":dbl, "P179":dbl, "P180":dbl, "P181":dbl, "P182":dbl, "P183":dbl, "P184":dbl, "P185":dbl, "P186":dbl, "P187":dbl, "P188":dbl, "P189":dbl, "P190":dbl, "P191":dbl, "P192":dbl, "P193":dbl, "P194":dbl, "P195":dbl, "P196":dbl, "P197":dbl, "P198":dbl, "P199":dbl, "P211":dbl, "P212":dbl, "P213":dbl, "P214":dbl, "P215":dbl, "P216":dbl, "P217":dbl, "P221":dbl, "P222":dbl, "P223":dbl, "P224":dbl, "P230":dbl, "P231":dbl, "P240":dbl, "P250":dbl, "P251":dbl}, "Parametri di configurazione":cluster{"C000":dbl, "C001":dbl, "C002":dbl, "C010":dbl, "C011":dbl, "C012":dbl, "C014":dbl, "C015":dbl, "C016":dbl, "C017":dbl, "C018":dbl, "C030":dbl, "C050":dbl, "C051":dbl, "C052":dbl, "C060":dbl, "C061":dbl, "C062":dbl, "C063":dbl, "C070":dbl, "C072":dbl, "C074":dbl, "C090":dbl, "C091":dbl, "C092":dbl, "C093":dbl, "C094":dbl, "C100":dbl, "C101":dbl, "C102":dbl, "C103":dbl, "C105":dbl, "C106":dbl, "C107":dbl, "C108":dbl, "C110":dbl, "C111":dbl, "C112":dbl, "C120":dbl, "C121":dbl, "C122":dbl, "C130":dbl, "C131":dbl, "C132":dbl, "C133":dbl, "C134":dbl, "C135":dbl, "C141":dbl, "C142":dbl, "C143":dbl, "C150":dbl, "C151":dbl, "C153":dbl, "C154":dbl, "C155":dbl, "C156":dbl, "C157":dbl, "C158":dbl, "C159":dbl, "C160":dbl, "C161":dbl, "C162":dbl, "C163":dbl, "C164":dbl, "C165":dbl, "C170":dbl}, "Codice allarme":dbl, "Comunicazione":bool}
  T30 = cluster{"Start da pulsantiera":bool, "Stop da pulsantiera":bool, "Reset da pulsantiera":bool, "Sistema OK":bool, "Collaudo abilitato":bool, "Potenza trifase abilitata":bool, "Potenza monofase abilitata":bool, "Potenza DC abilitata":bool, "Potenza DC ECC abilitata":bool, "Start alimentazione AC":bool, "Start alimentazione DC":bool, "Start DC eccitazione":bool, "Teleruttore WT abilitato":bool, "Teleruttore Resistomat abilitato":bool, "Teleruttore corto fasi":bool, "Ramo 1 resistomat":bool, "Ramo 2 resistomat":bool, "Ramo 3 resistomat":bool, "B1 Scelta linea elettrica 1":bool, "B1 Scelta linea elettrica 2":bool, "B1 Scelta linea elettrica 3":bool, "B1 Scelta linea elettrica 4":bool, "B1 Scelta linea elettrica 5":bool, "B2 Scelta linea elettrica 1":bool, "B2 Scelta linea elettrica 2":bool, "B2 Scelta linea elettrica 3":bool, "B2 Scelta linea elettrica 4":bool, "B2 Scelta linea elettrica 5":bool, "Rotore bloccato 1":bool, "Rotore bloccato 2":bool, "FRENO 1 abilitato":bool, "FRENO 1 run":bool, "FRENO 1 senso rotaz":bool, "FRENO 1 ctrl velocità":bool, "FRENO 2 abilitato":bool, "FRENO 2 run":bool, "FRENO 2 senso rotaz":bool, "FRENO 2 ctrl velocità":bool, "ALIM 1 abilitato":bool, "ALIM 1 run":bool, "ALIM 2 abilitato":bool, "ALIM 2 run":bool, "ALIM 3 abilitato":bool, "ALIM 3 run":bool, "FRENO 1 ctrl coppia":bool, "FRENO 2 ctrl coppia":bool, "FRENO 3 ctrl coppia":bool, "DI (logici) aggiuntivi impianto":cluster{"Solo freno abilitato":bool, "Carico resistivo abilitato":bool, "AFE+freno abilitato":bool, "Protezioni chiuse":bool, "Start potenza AFE":bool, "AFE in marcia":bool}, "Misura corrente diretta WT":bool, "Misura corrente sens ext":bool, "Sens ext abilitati":bool}
  T31 = enum32{"Invalid", "Standard", "Closed", "Hidden", "Minimized", "Maximized"}
  T32 = cluster{"Array of elements":cluster{"String":string, "variant":variant}[], "Single element":cluster{"String":string, "variant":variant}, "enque at\nopposite end (F)":bool, "no replications (F)":bool}
  T33 = typedef "SET ARRAY DO.ctl" = T34[]
  T34 = typedef "SET SINGLE DO.ctl" = cluster{"DO":T35, "Value":bool}
  T35 = typedef "DO List.ctl" = enum16{"OFF: ALL DO", "*ABILITA freno 1", "*ABILITA freno 2", "*ABILITA freno 3", "*START freno 1", "*START freno 2", "*START freno 3", "*STOP freno 1", "*STOP freno 3", "*STOP freno 2", "*Senso rot freno 1", "*Senso rot freno 2", "*Senso rot freno 3", "*Ctrl velocità freno 1", "*Ctrl velocità freno 2", "*Ctrl velocità freno 3", "*Ctrl coppia freno 1", "*Ctrl coppia freno 2", "*Ctrl coppia freno 3", "*ABILITA alimentatore 1", "*ABILITA alimentatore 2", "*ABILITA alimentatore 3", "*ABILITA alimentatore 4", "*START alimentatore 1", "*START alimentatore 2", "*START alimentatore 3", "*START alimentatore 4", "*STOP alimentatore 1", "*STOP alimentatore 2", "*STOP alimentatore 3", "*STOP alimentatore 4", "SENSO ROT alimentatore 1", "SENSO ROT alimentatore 2", "Abilita LEM 1000A", "Abilita LEM 300A", "Abilita sensori EXT WT", "B1 Seleziona linea 1", "B1 Seleziona linea 2", "B1 Seleziona linea 3", "B1 Seleziona linea 4", "B1 Seleziona linea 5", "B2 Seleziona linea 1", "B2 Seleziona linea 2", "B2 Seleziona linea 3", "B2 Seleziona linea 4", "B2 Seleziona linea 5", "*Reset allarmi", "*Start potenza AC", "*Stop potenza AC", "*Start potenza DC", "*Stop potenza DC", "*Start potenza DC eccit", "*Stop pontenza DC eccit", "Bypass res meter", "2nd canale res meter", "Enable res meter", "*Abilit teler ramo WT", "*Abil teler ramo princ Resit", "*Abil teler ramo 1 Resist", "*Abil teler ramo 2 Resist", "*Abil teler ramo 3 Resist", "*Abil cortocirc avvolgim", "*Controllo torsiometro B1", "*Controllo Torsiom B2", "*Scala torsiometro B1", "*Scala torsiometro B2", "*Collaudo in corso", "*Allarme presente", "Abilitazione elettroserratura", "Exit", "*Abilita collaudo", "*Abilita potenza trifase", "*Abilita potenza monofase", "*Abilita potenza DC", "*Abilita potenza DC eccit", "*Disabilita teleruttori potenza", "Set teleruttori prova a freddo", "Prova a freddo monofase", "Watchdog", "Forza DO PLC 3", "Forza DO PLC 2", "Forza DO PLC 1", "Forza DO cDAQ", "Scala 2000(T) 200(F) res meter", "Seleziona banco 1", "Seleziona banco 2", "Comando azionam in blocco", "Comando azionam reset", "Sensibilità freno 16 32 nm", "Reset Allarmi", "Carico res - Ramo 1", "Carico res - Ramo 2", "Carico res - Ramo 3", "Carico res - Ramo 4", "Carico res - Ramo 5", "Carico res - Ramo 6", "Carico res - Ramo 7", "Carico res - Ramo 8", "Carico res - Ramo 9", "Carico res - Ramo 10", "Carico res - Ramo 11", "Carico res - Start ventilatore", "Carico res - Stop ventilatore", "Abilita potenza solo freno", "Abilita AFE + freno trasc", "Abilita potenza carico resistivo", "Chiudi potenza AFE", "Apri potenza AFE", "Start AFE", "Config Banco2 TDE", "Misura diretto WT", "Ripristina centralina protezioni", "Abilita Scrittura Dati Keb", "Bench Selection(0-B1,1-B2)", "Select current mode", "Select torque mode", "Select speed mode", "Extenal alarm", "Enable Extenal program ", "Start ", "Stop", "Enable force mode", "Abilita linea 125 A", "Abilita linea 63 A", "Abilita linea 16 A", "Aum Tensione Variac", "Dim Tesnione Variac", "Abilita Ellecto Stractura", "Riprinto Emergenxe ", "Abilita Collaudo", "Disabilita Collaudo", "Abilita Ingresso Variac", "Abilita Uscita Variac", "Abilita ventilatore Variac"}
  T36 = cluster{"Message":string, "Message Data":variant}
  T37 = enum32{"Torque [Nm]", "Power [W]", "Speed [RPM]"}
  T38 = typedef "Comandi_Alimentatore.ctl" = cluster{"RIF 1":dbl, "RIF 2":dbl, "Status":cluster{"Ready":bool, "Running":bool, "Regulation":bool}, "Start\\stop":cluster{"Start":bool, "Stop":bool}, "PID RIF1":bool, "PID RIF2":bool, "Status ref":cluster{"RIF 1":dbl, "RIF 2":dbl}, "Abilita":cluster{"Abilita":bool}}
  T39 = cluster{"RIF 1":dbl, "RIF 2":dbl, "Abilitato":bool, "In marcia":bool, "Fine rampa RIF1":bool, "Fine rampa RIF2":bool, "Vstabile":bool, "F stabile":bool, "PID RIF1":bool, "PID RIF2":bool, "Alimentatore 1":T38}
  T40 = typedef "Stato inverter selezionato.ctl" = cluster{"Stato comandi freno":T41, "Stato":cluster{"rif C%":dbl, "rif vel%":dbl, "Controllo effettivo":enum32{"Torque [Nm]", "Power [W]", "Speed [RPM]"}, "Controllo desiderato":enum32{"Torque [Nm]", "Power [W]", "Speed [RPM]"}, "Fine rampa C":bool, "Fine rampa RPM":bool, "Senso rotaz":bool, "Start":bool, "C stabile":bool, "P stabile":bool, "RPM stabile":bool}}
  T41 = typedef "Comandi freno.ctl" = cluster{"Control":cluster{"Control Type":enum32{"Torque [Nm]", "Power [W]", "Speed [RPM]", "Corrente [A]"}, "Set":dbl, "Inverti senso di rotazione":bool}, "Start\\stop":cluster{"Start":bool, "STOP":bool}, "Status":cluster{"Ready":bool, "Running":bool, "Regulation":bool}, "PID":bool, "Abilita":cluster{"Abilita":bool}, "Status ref":cluster{"Torque":dbl, "Speed":dbl}}
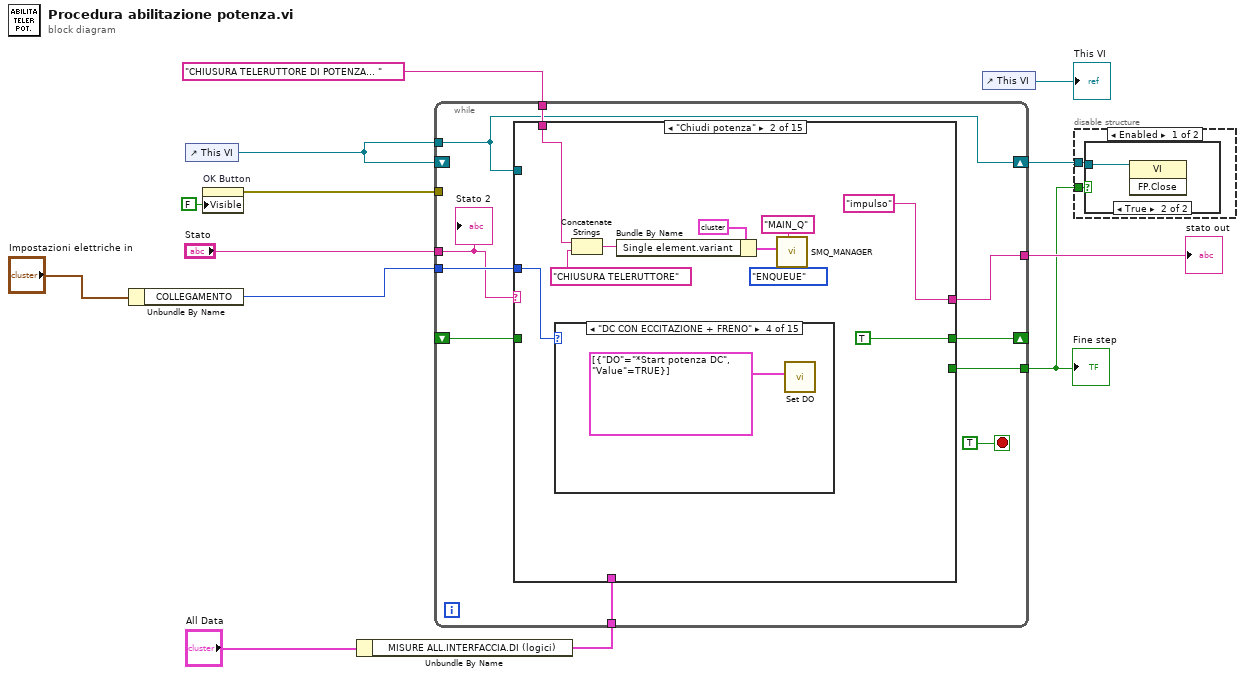
[diagram p0: block diagram]
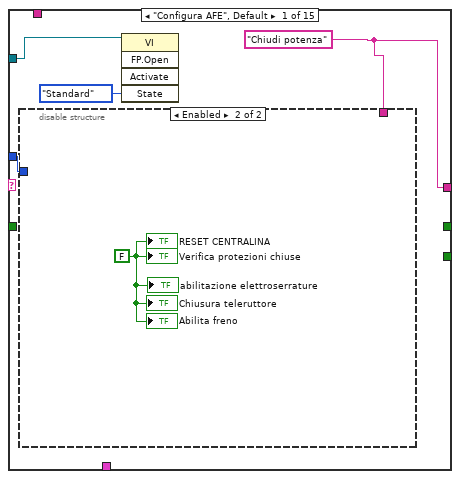
[diagram p4: hidden frame]
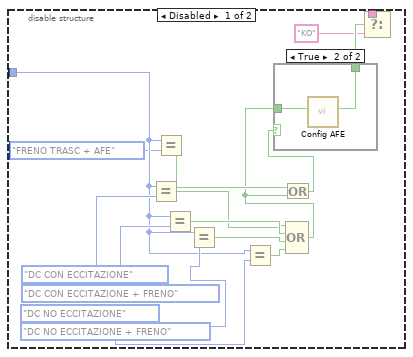
[diagram p5: hidden frame]
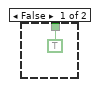
[diagram p6: hidden frame]
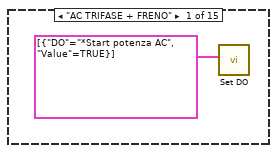
[diagram p7: hidden frame]
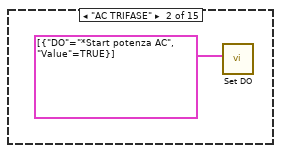
[diagram p8: hidden frame]
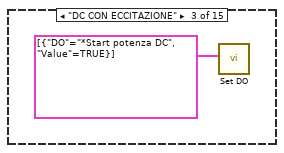
[diagram p9: hidden frame]
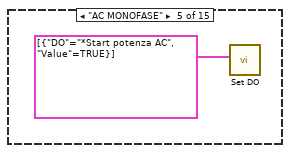
[diagram p10: hidden frame]
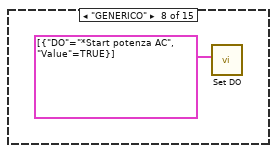
[diagram p13: hidden frame]
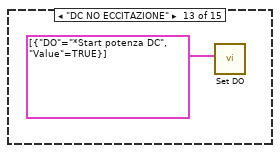
[diagram p18: hidden frame]
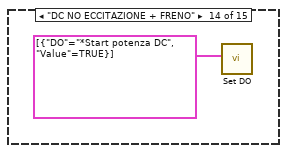
[diagram p19: hidden frame]
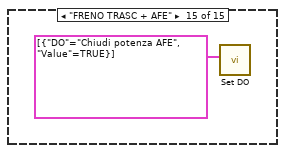
[diagram p20: hidden frame]
diagram:
  n1 = Unbundle By Name("Impostazioni elettriche in") -> ("COLLEGAMENTO"=w3:T2)
  n2 = control-ref of="This VI"() -> (w5:refnum<vi>)
  n3 = property on="OK Button" class="Bool (strict)"("Visible"=FALSE) -> (error out=w1:errorcluster)  [unwired: 2 in, 1 out]
  n4 = Unbundle By Name("All Data") -> ("MISURE ALL.INTERFACCIA.DI (logici)"=w8:T30)
  n5 = while {
    shift-right: [w22] -> _
    shift-left: _ -> [w21]
    tunnel: w3 -> [w20]
    tunnel: w8 -> [w19]
    tunnel: [w18] -> w7
    tunnel: "CHIUSURA TELERUTTORE DI POTENZA... " -> [w17]
    tunnel: "Stato" -> [w16]
    tunnel: [w15] -> w13
    shift-right: [w14] -> w6
    shift-left: w5 -> [_]
    tunnel: w5 -> [w14]
    tunnel: w1 -> [_]
    stop <- TRUE stop-if-true
    n6 = case shown="\"Chiudi potenza\"" w16 {
      selector: w16 -> [_ _ w68 _ w94 _ w110 w128 _ _ w147 _ w228 w261 w277]
      tunnel: [w26 "impulso" w67 "Attendi reset centralina" ("t") w95 "Attendi segnale protezioni chiuse" ("t") w111 w128 "Chiudi potenza" ("t") "wait" ("t") w150 "Attendi abilitazione" ("t") w222 w261 w277] -> w15
      tunnel: [_ TRUE _ TRUE _ TRUE _ _ _ TRUE _ TRUE _ _ w269] -> w22
      tunnel: w21 -> [_ _ w73 _ w99 _ w113 _ _ _ w155 _ w225 _ w269]
      tunnel: w20 -> [w27 w55 _ w75 _ _ _ _ _ w133 w151 w180 w219 _ _]
      tunnel: w19 -> [_ _ _ _ _ _ w114 _ _ _ w152 _ w230 _ _]
      tunnel: [_ _ _ _ _ _ _ "OK Button" _ _ _ _ _ TRUE ("Carico resistivo abilitato") TRUE ("Carico resistivo abilitato")] -> w18
      tunnel: w17 -> [_ w48 _ w79 _ _ _ w121 _ _ _ _ _ w253 w270]
      tunnel: w14 -> [w24 _ _ _ _ _ _ _ _ _ _ _ _ _ _]
      frame "Configura AFE", Default {
        w26 = "Chiudi potenza" ("t")
        n7 = disable-structure shown="Enabled" {
          disable-tunnel: w27 -> [w33 _]
          disable-tunnel: w26 -> [w28 _]
          frame Disabled {
            n8 = Equal?(x=w33, y=Collegamenti_elettrici."DC CON ECCITAZIONE" ("COLLEGAMENTO")) -> (x = y?=w34:bool)
            n9 = Equal?(x=w33, y=Collegamenti_elettrici."FRENO TRASC + AFE") -> (x = y?=w31:bool)
            n10 = Equal?(x=w33, y=Collegamenti_elettrici."DC CON ECCITAZIONE + FRENO" ("COLLEGAMENTO")) -> (x = y?=w35:bool)
            n11 = Equal?(x=w33, y=Collegamenti_elettrici."DC NO ECCITAZIONE" ("COLLEGAMENTO")) -> (x = y?=w36:bool)
            n12 = Equal?(x=w33, y=Collegamenti_elettrici."DC NO ECCITAZIONE + FRENO" ("COLLEGAMENTO")) -> (x = y?=w37:bool)
            n13 = Compound Arithmetic op=OR(w34, w35, w36, w37) -> (w30:bool)
            n14 = Or(x=w31, y=w30) -> (x .or. y?=w29:bool)
            n15 = case shown="True" w29 {
              tunnel: [TRUE ("OK") w46] -> w43
              tunnel: w30 -> [_ w45]
              frame False {
              }
              frame True {
                n16 = call "Config AFE.vi"("dc (T) altern (F)"=w45) -> ("OK"=w46:bool)  [unwired: 10 in]
              }
            }
            n17 = Select(t=w28, s=w43, f="KO") -> ()  [unwired: 1 out]
          }
          frame Enabled {
            w47 = FALSE ("Verifica protezioni chiuse")
            "Verifica protezioni chiuse" <- w47
            "abilitazione elettroserrature" <- w47
            "Chiusura teleruttore" <- w47
            "RESET CENTRALINA" <- w47
            "Abilita freno" <- w47
          }
        }
        n18 = invoke class="VI" method="FP.Open"(reference=w24, "State"=T31."Standard") -> ()  [unwired: 3 in, 5 out]
      }
      frame "Chiudi potenza" {
        n19 = case shown="\"DC CON ECCITAZIONE + FRENO\"" w55 {
          frame "AC TRIFASE + FRENO" {
            n20 = call "Set DO.vi"("Cluster SET DO"=T33 [{"DO"=enum."*Start potenza AC", "Value"=TRUE}]) -> ()  [unwired: 10 in, 1 out]
          }
          frame "AC TRIFASE" {
            n21 = call "Set DO.vi"("Cluster SET DO"=T33 [{"DO"=enum."*Start potenza AC", "Value"=TRUE}]) -> ()  [unwired: 10 in, 1 out]
          }
          frame "DC CON ECCITAZIONE" {
            n22 = call "Set DO.vi"("Cluster SET DO"=T33 [{"DO"=enum."*Start potenza DC", "Value"=TRUE}]) -> ()  [unwired: 10 in, 1 out]
          }
          frame "DC CON ECCITAZIONE + FRENO" {
            n23 = call "Set DO.vi"("Cluster SET DO"=T33 [{"DO"=enum."*Start potenza DC", "Value"=TRUE}]) -> ()  [unwired: 10 in, 1 out]
          }
          frame "AC MONOFASE" {
            n24 = call "Set DO.vi"("Cluster SET DO"=T33 [{"DO"=enum."*Start potenza AC", "Value"=TRUE}]) -> ()  [unwired: 10 in, 1 out]
          }
          frame "SOLO FRENO" {
          }
          frame "CARICO RESISTIVO" {
          }
          frame "GENERICO" {
            n25 = call "Set DO.vi"("Cluster SET DO"=T33 [{"DO"=enum."*Start potenza AC", "Value"=TRUE}]) -> ()  [unwired: 10 in, 1 out]
          }
          frame "SOLO ACQUISITORE" {
          }
          frame "SCORTA 4" {
          }
          frame "SCORTA 5" {
          }
          frame "SCORTA 6" {
          }
          frame "DC NO ECCITAZIONE" {
            n26 = call "Set DO.vi"("Cluster SET DO"=T33 [{"DO"=enum."*Start potenza DC", "Value"=TRUE}]) -> ()  [unwired: 10 in, 1 out]
          }
          frame "DC NO ECCITAZIONE + FRENO" {
            n27 = call "Set DO.vi"("Cluster SET DO"=T33 [{"DO"=enum."*Start potenza DC", "Value"=TRUE}]) -> ()  [unwired: 10 in, 1 out]
          }
          frame "FRENO TRASC + AFE" {
            n28 = call "Set DO.vi"("Cluster SET DO"=T33 [{"DO"=enum."Chiudi potenza AFE", "Value"=TRUE}]) -> ()  [unwired: 10 in, 1 out]
          }
        }
        n29 = Concatenate Strings(w48, "CHIUSURA TELERUTTORE") -> (w53:string)
        n30 = Bundle By Name(cluster=T32 {"Array of elements"=[], "Single element"={"String"="AGGIORNA STATUS", "variant"=variant}, "enque at\nopposite end (F)"=FALSE, "no replications (F)"=FALSE} ("Enqueue cluster"), "Single element.variant"=w53) -> (w52:T32)
        n31 = call <userlib>:"SMQ_MANAGER.vi"("Function"=enum16{"INITIALIZE", "ENQUEUE", "STOP ALL"}."ENQUEUE", "Queue name"="MAIN_Q", "Enqueue cluster"=w52) -> ()  [unwired: 8 in, 1 out]
      }
      frame "impulso" {
        n32 = call "Elapsed Time4"("Time Target (s)"=2.0, "Reset"=w73, "Auto Reset"=FALSE) -> ("Time has Elapsed"=w70:bool)  [unwired: 9 in, 7 out]
        n33 = Select(t="Chiudi potenza off", s=w70, f=w68) -> (s? t:f=w67:string)
      }
      frame "Alza reset centralina" {
        n34 = case shown="\"SOLO FRENO\"" w75 {
          tunnel: [_ TRUE _ _ TRUE _ TRUE TRUE TRUE _ _ _ _ _ _] -> w74
          frame "AC TRIFASE", Default {
          }
          frame "AC TRIFASE + FRENO" {
          }
          frame "AC MONOFASE" {
          }
          frame "DC CON ECCITAZIONE" {
          }
          frame "DC CON ECCITAZIONE + FRENO" {
          }
          frame "DC NO ECCITAZIONE" {
          }
          frame "DC NO ECCITAZIONE + FRENO" {
          }
          frame "FRENO TRASC + AFE" {
          }
          frame "SOLO FRENO" {
          }
          frame "CARICO RESISTIVO" {
          }
          frame "GENERICO" {
          }
          frame "SOLO ACQUISITORE" {
          }
          frame "SCORTA 4" {
          }
          frame "SCORTA 5" {
          }
          frame "SCORTA 6" {
          }
        }
        n35 = Concatenate Strings(w79, "VERIFICA CHIUSURA PROTEZIONI") -> (w84:string)
        n36 = Bundle By Name(cluster=T32 {"Array of elements"=[], "Single element"={"String"="AGGIORNA STATUS", "variant"=variant}, "enque at\nopposite end (F)"=FALSE, "no replications (F)"=FALSE} ("Enqueue cluster"), "Single element.variant"=w84) -> (w83:T32)
        n37 = property on="Abilita freno" class="Bool (strict)"("Visible"=w74) -> ()  [unwired: 2 in, 2 out]
        n38 = local write "OK Button"(FALSE ("OK Button")) -> ()
        n39 = call <userlib>:"SMQ_MANAGER.vi"("Function"=enum16{"INITIALIZE", "ENQUEUE", "STOP ALL"}."ENQUEUE", "Queue name"="MAIN_Q", "Enqueue cluster"=w83) -> ()  [unwired: 8 in, 1 out]
        n40 = property on="OK Button" class="Bool (strict)"("Visible"=FALSE) -> ()  [unwired: 2 in, 2 out]
        n41 = property on="String" class="Str"("Visible"=FALSE) -> ()  [unwired: 2 in, 2 out]
        n42 = call "Set DO.vi"("Cluster SET DO"=T33 [{"DO"=enum."Ripristina centralina protezioni", "Value"=TRUE}]) -> ()  [unwired: 10 in, 1 out]
      }
      frame "Attendi reset centralina" {
        n43 = call "Elapsed Time"("Time Target (s)"=1.0, "Reset"=w99, "Auto Reset"=FALSE) -> ("Time has Elapsed"=w98:bool)  [unwired: 9 in, 7 out]
        n44 = Select(t="Abbassa reset centralina", s=w98, f=w94) -> (s? t:f=w95:string)
      }
      frame "Abbassa reset centralina" {
        n45 = local write "RESET CENTRALINA"(TRUE ("RESET CENTRALINA")) -> ()
        n46 = call "Set DO.vi"("Cluster SET DO"=T33 [{"DO"=enum."Ripristina centralina protezioni", "Value"=FALSE}]) -> ()  [unwired: 10 in, 1 out]
      }
      frame "Attendi segnale protezioni chiuse" {
        n47 = Unbundle By Name(w114) -> ("DI (logici) aggiuntivi impianto.Protezioni chiuse"=w105:bool)
        n48 = call "Elapsed Time2"("Time Target (s)"=5.0, "Reset"=w113) -> ("Time has Elapsed"=w112:bool)  [unwired: 10 in, 7 out]
        n49 = local write "Verifica protezioni chiuse"(w105) -> ()
        n50 = Select(t="Elettroserrature aperte", s=w112, f=w110) -> (s? t:f=w109:string)
        n51 = Select(t="Abilita elettroserratura", s=w105, f=w109) -> (s? t:f=w111:string)
      }
      frame "Elettroserrature aperte" {
        n52 = Concatenate Strings(w121, "KO: CHIUDERE LE PROTEZIONI") -> (w126:string)
        n53 = Bundle By Name(cluster=T32 {"Array of elements"=[], "Single element"={"String"="AGGIORNA STATUS", "variant"=variant}, "enque at\nopposite end (F)"=FALSE, "no replications (F)"=FALSE} ("Enqueue cluster"), "Single element.variant"=w126) -> (w125:T32)
        n54 = property on="OK Button" class="Bool (strict)"("Visible"=TRUE, "Blinking"=FALSE) -> ()  [unwired: 2 in, 2 out]
        n55 = call <userlib>:"SMQ_MANAGER.vi"("Function"=enum16{"INITIALIZE", "ENQUEUE", "STOP ALL"}."ENQUEUE", "Queue name"="MAIN_Q", "Enqueue cluster"=w125) -> ()  [unwired: 8 in, 1 out]
        n56 = property on="String" class="Str"("Visible"=TRUE) -> ()  [unwired: 2 in, 2 out]
        n57 = call "Set DO.vi"("Cluster SET DO"=T33 [{"DO"=enum."Ripristina centralina protezioni", "Value"=FALSE}]) -> ()  [unwired: 10 in, 1 out]
        "String" <- "ATTENZIONE: LE PROTEZIONI RISULTANO APERTE. CHIUDERLE E RIPROVARE." ("String")
      }
      frame "Abilita elettroserratura" {
        n58 = local write "abilitazione elettroserrature"(TRUE ("abilitazione elettroserrature")) -> ()
        n59 = call "Set DO.vi"("Cluster SET DO"=T33 [{"DO"=enum."Abilitazione elettroserratura", "Value"=TRUE}]) -> ()  [unwired: 10 in, 1 out]
      }
      frame "Chiudi potenza off" {
        n60 = case shown="\"AC TRIFASE + FRENO\"" w133 {
          frame "AC TRIFASE + FRENO" {
            n61 = call "Set DO.vi"("Cluster SET DO"=T33 [{"DO"=enum."*Start potenza AC", "Value"=FALSE}]) -> ()  [unwired: 10 in, 1 out]
          }
          frame "AC TRIFASE" {
            n62 = call "Set DO.vi"("Cluster SET DO"=T33 [{"DO"=enum."*Start potenza AC", "Value"=FALSE}]) -> ()  [unwired: 10 in, 1 out]
          }
          frame "DC CON ECCITAZIONE" {
            n63 = call "Set DO.vi"("Cluster SET DO"=T33 [{"DO"=enum."*Start potenza DC", "Value"=FALSE}]) -> ()  [unwired: 10 in, 1 out]
          }
          frame "DC CON ECCITAZIONE + FRENO" {
            n64 = call "Set DO.vi"("Cluster SET DO"=T33 [{"DO"=enum."*Start potenza DC", "Value"=FALSE}]) -> ()  [unwired: 10 in, 1 out]
          }
          frame "AC MONOFASE" {
            n65 = call "Set DO.vi"("Cluster SET DO"=T33 [{"DO"=enum."*Start potenza AC", "Value"=FALSE}]) -> ()  [unwired: 10 in, 1 out]
          }
          frame "SOLO FRENO" {
          }
          frame "CARICO RESISTIVO" {
          }
          frame "GENERICO" {
            n66 = call "Set DO.vi"("Cluster SET DO"=T33 [{"DO"=enum."*Start potenza AC", "Value"=FALSE}]) -> ()  [unwired: 10 in, 1 out]
          }
          frame "SOLO ACQUISITORE" {
          }
          frame "SCORTA 4" {
          }
          frame "SCORTA 5" {
          }
          frame "SCORTA 6" {
          }
          frame "DC NO ECCITAZIONE" {
            n67 = call "Set DO.vi"("Cluster SET DO"=T33 [{"DO"=enum."*Start potenza DC", "Value"=FALSE}]) -> ()  [unwired: 10 in, 1 out]
          }
          frame "DC NO ECCITAZIONE + FRENO" {
            n68 = call "Set DO.vi"("Cluster SET DO"=T33 [{"DO"=enum."*Start potenza DC", "Value"=FALSE}]) -> ()  [unwired: 10 in, 1 out]
          }
          frame "FRENO TRASC + AFE" {
            n69 = call "Set DO.vi"("Cluster SET DO"=T33 [{"DO"=enum."Chiudi potenza AFE", "Value"=FALSE}]) -> ()  [unwired: 10 in, 1 out]
          }
        }
      }
      frame "wait" {
        n70 = case shown="\"AC TRIFASE + FRENO\"" w151 {
          tunnel: [w157 w162 w164 w166 w167 TRUE ("Start potenza AFE") w170 w172 _ _ _ _ w174 w176 w178] -> w145
          tunnel: w152 -> [w156 w161 w163 w165 w168 _ w171 w173 _ _ _ _ w175 w177 w179]
          frame "AC TRIFASE + FRENO" {
            n71 = disable-structure shown="Disabled" {
              disable-tunnel: [w159 TRUE] -> w157
              disable-tunnel: w156 -> [w158 _]
              frame Disabled {
                n72 = Unbundle By Name(w158) -> ("Start alimentazione AC"=w159:bool)
              }
              frame Enabled {
              }
            }
          }
          frame "DC CON ECCITAZIONE" {
            (unwired) FALSE
            n73 = Unbundle By Name(w161) -> ("Start alimentazione DC"=w162:bool)
          }
          frame "DC CON ECCITAZIONE + FRENO" {
            (unwired) TRUE
            n74 = Unbundle By Name(w163) -> ("Start alimentazione DC"=w164:bool)
          }
          frame "AC TRIFASE" {
            (unwired) FALSE
            n75 = Unbundle By Name(w165) -> ("Start alimentazione AC"=w166:bool)
          }
          frame "AC MONOFASE" {
            n76 = Unbundle By Name(w168) -> ("Start alimentazione AC"=w167:bool)
          }
          frame "SOLO FRENO" {
          }
          frame "CARICO RESISTIVO" {
            (unwired) FALSE
            n77 = Unbundle By Name(w171) -> ("DI (logici) aggiuntivi impianto.Carico resistivo abilitato"=w170:bool)
          }
          frame "GENERICO" {
            (unwired) FALSE
            n78 = Unbundle By Name(w173) -> ("Start alimentazione AC"=w172:bool)
          }
          frame "SOLO ACQUISITORE" {
          }
          frame "SCORTA 4" {
          }
          frame "SCORTA 5" {
          }
          frame "SCORTA 6" {
          }
          frame "DC NO ECCITAZIONE" {
            n79 = Unbundle By Name(w175) -> ("Potenza DC abilitata"=w174:bool)
          }
          frame "DC NO ECCITAZIONE + FRENO" {
            (unwired) TRUE
            n80 = Unbundle By Name(w177) -> ("Potenza DC abilitata"=w176:bool)
          }
          frame "FRENO TRASC + AFE" {
            (unwired) TRUE
            n81 = Unbundle By Name(w179) -> ("DI (logici) aggiuntivi impianto.Start potenza AFE"=w178:bool)
          }
        }
        n82 = call "Elapsed Time3"("Time Target (s)"=5.0, "Reset"=w155, "Auto Reset"=FALSE) -> ("Time has Elapsed"=w149:bool)  [unwired: 9 in, 7 out]
        n83 = local write "Chiusura teleruttore"(w145) -> ()
        n84 = Select(t="KO", s=w149, f=w147) -> (s? t:f=w146:string)
        n85 = Select(t="Abilita freno alimentatore", s=w145, f=w146) -> (s? t:f=w150:string)
      }
      frame "Abilita freno alimentatore" {
        n86 = case shown="\"AC TRIFASE + FRENO\"" w180 {
          frame "AC TRIFASE", Default {
            n87 = global read "Stato alimentatore 1.vi" "Stato alimentatore 1"() -> (w191:T39)
            n88 = Unbundle By Name(w191) -> ("Alimentatore 1"=w190:T38)
            n89 = Bundle By Name(cluster=w190, "Abilita.Abilita"=TRUE ("Alimentatore 1.Command.Start")) -> (w189:T38)
            n90 = Obtain Queue(name (unnamed)="ALIMENTATORE 1", element data type=T36 {"Message"="", "Message Data"=variant} ("Message Cluster")) -> (queue out=w188:refnum<queue>)  [unwired: 3 in, 2 out]
            n91 = Bundle By Name(cluster=cluster{"Status":string, "variant":variant} {"Status"="AGGIORNA COMANDI ALIMENTATORE", "variant"=variant}, "variant"=w189) -> (w187:cluster{"Status":string, "variant":variant})
            n92 = Enqueue Element(queue=w188, element=w187) -> ()  [unwired: 2 in, 3 out]
          }
          frame "AC TRIFASE + FRENO" {
            n93 = global read "Stato alimentatore 1.vi" "Stato alimentatore 1"() -> (w200:T39)
            n94 = global read "Stato comandi freno.vi" "Stato inverter"() -> (w202:T40)
            n95 = Unbundle By Name(w202) -> ("Stato comandi freno"=w201:T41)
            n96 = Unbundle By Name(w200) -> ("Alimentatore 1"=w199:T38)
            n97 = Bundle By Name(cluster=w201, "Abilita.Abilita"=TRUE ("Stato comandi freno.Abilita.Abilita")) -> (w205:T41)
            n98 = Bundle By Name(cluster=w199, "Abilita.Abilita"=TRUE ("Alimentatore 1.Command.Start")) -> (w198:T38)
            n99 = Obtain Queue(name (unnamed)="FRENI", element data type=T36 {"Message"="", "Message Data"=variant} ("Message Cluster")) -> (queue out=w206:refnum<queue>)  [unwired: 3 in, 2 out]
            n100 = Obtain Queue(name (unnamed)="ALIMENTATORE 1", element data type=T36 {"Message"="", "Message Data"=variant} ("Message Cluster")) -> (queue out=w197:refnum<queue>)  [unwired: 3 in, 2 out]
            n101 = Bundle By Name(cluster=cluster{"Status":string, "variant":variant} {"Status"="AGGIORNA COMANDI ALIMENTATORE", "variant"=variant}, "variant"=w198) -> (w196:cluster{"Status":string, "variant":variant})
            n102 = Bundle By Name(cluster=cluster{"Status":string, "variant":variant} {"Status"="AGGIORNA COMANDI FRENO", "variant"=variant}, "variant"=w205) -> (w209:cluster{"Status":string, "variant":variant})
            n103 = Enqueue Element(queue=w197, element=w196) -> ()  [unwired: 2 in, 3 out]
            n104 = Enqueue Element(queue=w206, element=w209) -> ()  [unwired: 2 in, 3 out]
          }
          frame "AC MONOFASE" {
          }
          frame "DC CON ECCITAZIONE" {
          }
          frame "DC CON ECCITAZIONE + FRENO" {
          }
          frame "DC NO ECCITAZIONE" {
          }
          frame "DC NO ECCITAZIONE + FRENO" {
          }
          frame "FRENO TRASC + AFE" {
          }
          frame "SOLO FRENO" {
            n105 = global read "Stato comandi freno.vi" "Stato inverter"() -> (w215:T40)
            n106 = Unbundle By Name(w215) -> ("Stato comandi freno"=w214:T41)
            n107 = Bundle By Name(cluster=w214, "Abilita.Abilita"=TRUE ("Stato comandi freno.Abilita.Abilita")) -> (w216:T41)
            n108 = Obtain Queue(name (unnamed)="FRENI", element data type=T36 {"Message"="", "Message Data"=variant} ("Message Cluster")) -> (queue out=w217:refnum<queue>)  [unwired: 3 in, 2 out]
            n109 = Bundle By Name(cluster=cluster{"Status":string, "variant":variant} {"Status"="AGGIORNA COMANDI FRENO", "variant"=variant}, "variant"=w216) -> (w218:cluster{"Status":string, "variant":variant})
            n110 = Enqueue Element(queue=w217, element=w218) -> ()  [unwired: 2 in, 3 out]
          }
          frame "CARICO RESISTIVO" {
          }
          frame "GENERICO" {
          }
          frame "SOLO ACQUISITORE" {
          }
          frame "SCORTA 4" {
          }
          frame "SCORTA 5" {
          }
          frame "SCORTA 6" {
          }
        }
      }
      frame "Attendi abilitazione" {
        n111 = case shown="\"AC TRIFASE + FRENO\"" w219 {
          tunnel: w230 -> [w234 w240 _ _ _ _ _ _ w252 _ _ _ _ _ _]
          tunnel: [w233 w239 _ _ _ _ _ _ w250 _ _ _ _ _ _] -> w229
          frame "AC TRIFASE", Default {
            n112 = Unbundle By Name(w234) -> ("ALIM 1 abilitato"=w232:bool, "ALIM 2 abilitato"=w231:bool)
            n113 = Or(x=w232, y=w231) -> (x .or. y?=w233:bool)
          }
          frame "AC TRIFASE + FRENO" {
            n114 = Unbundle By Name(w240) -> ("FRENO 2 abilitato"=w237:bool, "FRENO 1 abilitato"=w236:bool, "ALIM 1 abilitato"=w238:bool, "ALIM 2 abilitato"=w235:bool)
            n115 = disable-structure shown="Enabled" {
              disable-tunnel: [w247 TRUE] -> w239
              disable-tunnel: w238 -> [w246 _]
              disable-tunnel: w237 -> [w244 _]
              disable-tunnel: w236 -> [w243 _]
              disable-tunnel: w235 -> [w241 _]
              frame Disabled {
                n116 = Or(x=w244, y=w243) -> (x .or. y?=w245:bool)
                n117 = Or(x=w246, y=w241) -> (x .or. y?=w242:bool)
                n118 = And(x=w245, y=w242) -> (x .and. y?=w247:bool)
              }
              frame Enabled {
              }
            }
          }
          frame "AC MONOFASE" {
          }
          frame "DC CON ECCITAZIONE" {
          }
          frame "DC CON ECCITAZIONE + FRENO" {
          }
          frame "DC NO ECCITAZIONE" {
          }
          frame "DC NO ECCITAZIONE + FRENO" {
          }
          frame "FRENO TRASC + AFE" {
          }
          frame "SOLO FRENO" {
            n119 = Unbundle By Name(w252) -> ("FRENO 1 abilitato"=w251:bool, "FRENO 2 abilitato"=w249:bool)
            n120 = Or(x=w251, y=w249) -> (x .or. y?=w250:bool)
          }
          frame "CARICO RESISTIVO" {
          }
          frame "GENERICO" {
          }
          frame "SOLO ACQUISITORE" {
          }
          frame "SCORTA 4" {
          }
          frame "SCORTA 5" {
          }
          frame "SCORTA 6" {
          }
        }
        n121 = call "Elapsed Time5"("Time Target (s)"=10.0, "Reset"=w225, "Auto Reset"=FALSE) -> ("Time has Elapsed"=w224:bool)  [unwired: 9 in, 7 out]
        n122 = local write "Abilita freno"(w229) -> ()
        n123 = Select(t="OK", s=w229, f=w228) -> (s? t:f=w223:string)
        n124 = Select(t="KO", s=w224, f=w223) -> (s? t:f=w222:string)
      }
      frame "KO" {
        (unwired) "KO" ("t")
        n125 = Concatenate Strings(w253, "KO.") -> (w258:string)
        n126 = Bundle By Name(cluster=T32 {"Array of elements"=[], "Single element"={"String"="AGGIORNA STATUS", "variant"=variant}, "enque at\nopposite end (F)"=FALSE, "no replications (F)"=FALSE} ("Enqueue cluster"), "Single element.variant"=w258) -> (w257:T32)
        n127 = global write "Global allarmi procedure.vi" "Allarme Start potenza"(TRUE ("Allarme Abilita potenza")) -> ()
        n128 = call <userlib>:"SMQ_MANAGER.vi"("Function"=enum16{"INITIALIZE", "ENQUEUE", "STOP ALL"}."ENQUEUE", "Queue name"="MAIN_Q", "Enqueue cluster"=w257) -> ()  [unwired: 8 in, 1 out]
      }
      frame "OK" {
        n129 = Concatenate Strings(w270, "OK.") -> (w275:string)
        n130 = Bundle By Name(cluster=T32 {"Array of elements"=[], "Single element"={"String"="AGGIORNA STATUS", "variant"=variant}, "enque at\nopposite end (F)"=FALSE, "no replications (F)"=FALSE} ("Enqueue cluster"), "Single element.variant"=w275) -> (w274:T32)
        n131 = Bundle By Name(cluster=cluster{"Status":string, "variant":variant} {"Status"="Set tipo controllo", "variant"=variant}, "variant"=T37."Torque [Nm]" ("Control Type")) -> (w264:cluster{"Status":string, "variant":variant})
        n132 = Obtain Queue(name (unnamed)="FRENI", element data type=T36 {"Message"="", "Message Data"=variant} ("Message Cluster")) -> (queue out=w268:refnum<queue>)  [unwired: 3 in, 2 out]
        n133 = call <userlib>:"SMQ_MANAGER.vi"("Function"=enum16{"INITIALIZE", "ENQUEUE", "STOP ALL"}."ENQUEUE", "Queue name"="MAIN_Q", "Enqueue cluster"=w274) -> ()  [unwired: 8 in, 1 out]
        n134 = Enqueue Element(queue=w268, element=w264) -> ()  [unwired: 2 in, 3 out]
      }
    }
    "Stato 2" <- w16
  }
  "stato out" <- w13
  "Fine step" <- w7
  n135 = control-ref of="This VI"() -> (→"This VI":refnum<vi>)
  n136 = disable-structure shown="Enabled" {
    disable-tunnel: w7 -> [w280 _]
    disable-tunnel: w6 -> [w279 _]
    frame Enabled {
      n137 = case shown="True" w280 {
        tunnel: w279 -> [_ w281]
        frame False {
        }
        frame True {
          n138 = invoke class="VI" method="FP.Close"(reference=w281) -> ()  [unwired: 2 in, 3 out]
        }
      }
    }
    frame Disabled {
    }
  }
